vi "Get Data.vi"(3 "Data":T1 {"Уд. сопротивление" format="%#.3f"; "Сопротивление" format="%#.3f"; "Диаметр" format="%#.3f"; "Длина" format="%#.3f"}) -> (0 "Array of Data":string[](array[string]), 1 "Array of Headers":string[](array[string]))   [LabVIEW 2023, in "Registration.lvclass"]
uses:
  Registration.lvclass
  rqp_Data.ctl
panel:
  out "error out":errorcluster
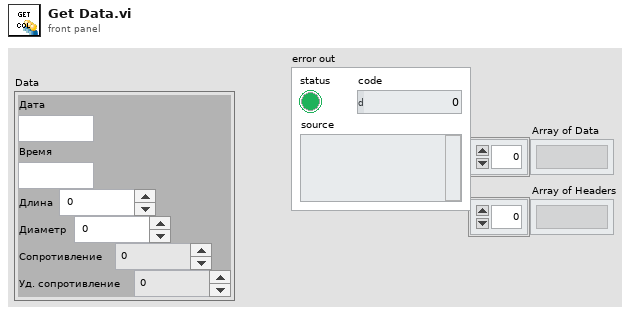
[diagram p1: front panel]
types:
  T1 = typedef "Registration.lvclass/rqp_Data.ctl" = cluster{"Дата":string, "Время":string, "Длина":dbl, "Диаметр":dbl, "Сопротивление":dbl, "Уд. сопротивление":dbl}
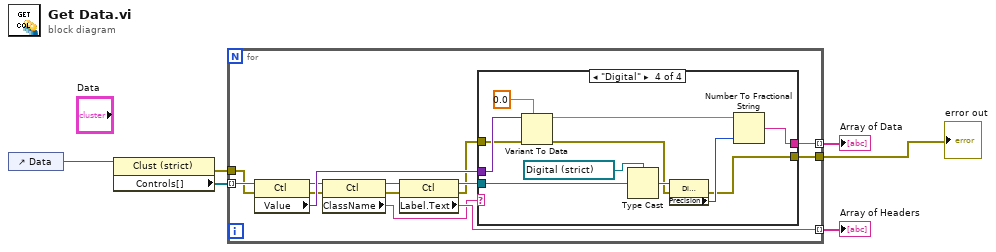
[diagram p0: block diagram]
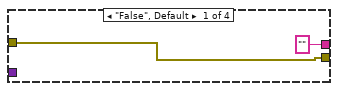
[diagram p2: hidden frame]
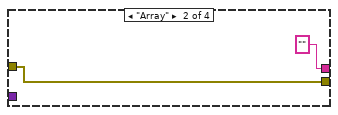
[diagram p3: hidden frame]
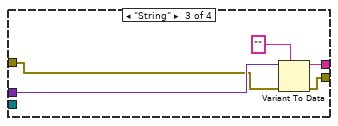
[diagram p4: hidden frame]
diagram:
  n1 = control-ref of="Data"() -> (w3:refnum<vi>)
  n2 = property class="Clust (strict)"(reference=w3) -> (error out=w2:errorcluster, "Controls[]"=w6:refnum<vi>[])  [unwired: 1 in, 1 out]
  n3 = for {
    tunnel: w6 -> [w19] mode=indexing
    tunnel: [w16] -> w5 mode=indexing
    tunnel: [w14] -> w4 mode=indexing
    tunnel: w2 -> [w11]
    tunnel: [w7] -> w1
    n4 = property class="Ctl"(reference=w19, error in=w11) -> (reference out=w17:refnum<vi>, error out=w10:errorcluster, "Value"=w18:variant)
    n5 = property class="Ctl"(reference=w17, error in=w10) -> (reference out=w15:refnum<vi>, error out=w9:errorcluster, "ClassName"=w13:string)
    n6 = property class="Ctl"(reference=w15, error in=w9) -> (reference out=w12:refnum<vi>, error out=w8:errorcluster, "Label.Text"=w14:string)
    n7 = case shown="\"Digital\"" w13 {
      tunnel: w18 -> [_ _ w27 w39]
      tunnel: ["" "" w26 w36] -> w16
      tunnel: w12 -> [_ _ _ w35]
      tunnel: w8 -> [w20 w22 w25 w31]
      tunnel: [w20 w22 w24 w29] -> w7
      frame "False", Default {
      }
      frame "Array" {
      }
      frame "String" {
        n8 = Variant To Data(error in=w25, type="", Variant=w27) -> (data=w26:string, error out=w24:errorcluster)
      }
      frame "Digital" {
        n9 = Variant To Data(error in=w31, type=0.0, Variant=w39) -> (data=w37:dbl, error out=w30:errorcluster)
        n10 = Type Cast(type=refnum<vi> refnum ("Numeric"), x=w35) -> (*(type *) &x=w33:refnum<vi>)
        n11 = property class="DigNum (strict)"(reference=w33, error in=w30) -> (error out=w29:errorcluster, "Precision"=w32:u8)  [unwired: 1 out]
        n12 = Number To Fractional String(number=w37, precision (6)=w32) -> (F-format string=w36:string)  [unwired: 2 in]
      }
    }
  }
  "Array of Data" <- w5
  "Array of Headers" <- w4
  "error out" <- w1
